vi "Function Generator Sweep.vi"(1 "Action":T3=enum."Identify", 2 "Parameters":variant) -> (6 "Output":variant, 7 "Stop":bool)   [LabVIEW 2020]
doc: "This VI reads a single reading from a Keithley 2001 multimeter. The stop boolean is always false. If no reading is obtained a single zero is returned.\nScott Hannahs, NHMFL-FSU, Nov 1993"
uses:
  Sub Controls/Instrument Actions.ctl
  Sub Controls/Instrument Match.ctl
  Sub Controls/Public.ctl
  Sub Controls/Scan Output.ctl
  Sub Controls/Instrument IDN.ctl
  Sub Controls/User Event Command.ctl
  <vilib>/Instr/_visa.llb/VISA GPIB Control REN Mode.ctl
panel:
  in  "Index":i32
  in  "Wait After Setting":dbl=5.0 format="%<%M:%S>t"
  in  "Mapping":bool
  in  "Time":dbl=1200.0 format="%<%H:%M:%S>t"
  in  "End Value":dbl=20.0
  in  "Start Value":dbl=1.0
  in  "Mode":bool
  out "Title":string
  in  "Public":T1
  in  "Address":u16(ring)
  out "Model":string
  in  "Instruments":T2[](array[typedef])=[{"Model"="DS360", "Manufacturer"="StanfordResearchSystems", "Term Character"="", "Wait Time (mS)"=0, "Wait for SRQ"=FALSE, "Type"="Func. Gen."}, {"Model"="SR830", "Manufacturer"="Stanford_Research_Systems", "Term Character"="", "Wait Time (mS)"=0, "Wait for SRQ"=FALSE, "Type"="Func. Gen."}, {"Model"="SR865A*", "Manufacturer"="Stanford_Research_Systems", "Term Character"="", "Wait Time (mS)"=0, "Wait for SRQ"=FALSE, "Type"="Func. Gen."}, {"Model"="SR860", "Manufacturer"="Stanford_Research_Systems", "Term Character"="", "Wait Time (mS)"=0, "Wait for SRQ"=FALSE, "Type"="Func. Gen."}]
  out "Measurement":dbl[](array[numeric]) format="%^_7e"
  in  "VISA resource name":refnum<visa-resource-name>
  # "Term Char"
  # "Wait Time (mS)"
  # "Wait for SRQ?"
  # "Type"
  # "Manufacturer"
  # "Model"
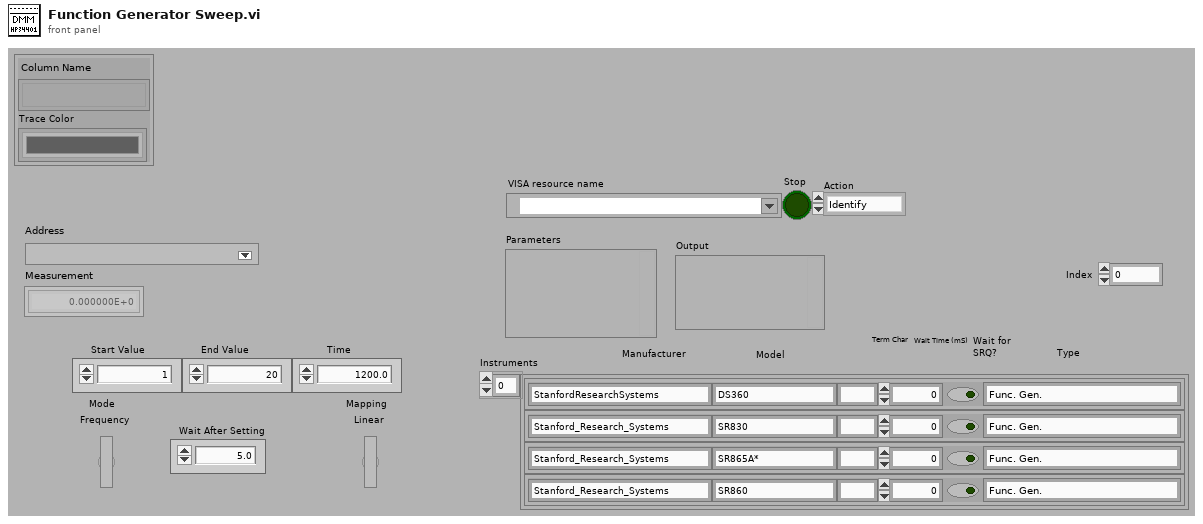
[diagram p1: front panel]
types:
  T1 = typedef "Public.ctl" = cluster{"Column Name":string[], "Trace Color":u32[]}
  T2 = typedef "Instrument Match.ctl" = cluster{"Model":string, "Manufacturer":string, "Term Character":string, "Wait Time (mS)":u32, "Wait for SRQ":bool, "Type":string}
  T3 = typedef "Instrument Actions.ctl" = enum16{"Scan", "Identify", "New", "Configure", "Initialize", "Test", "Read", "Close"}
  T4 = typedef "Scan Output.ctl" = cluster{"Manufacturer":string, "Model":string, "Info":string, "Revision":string, "error out":errorcluster}
  T5 = typedef "Instrument IDN.ctl" = cluster{"VISA Address":string, "Status":u16, "Manufacturer":string, "Model":string, "Info":string, "Info 2":string, "Misc Data":variant}
  T6 = typedef "User Event Command.ctl" = enum32{"Stop Config"}
  T7 = typedef "VISA GPIB Control REN Mode.ctl" = u16
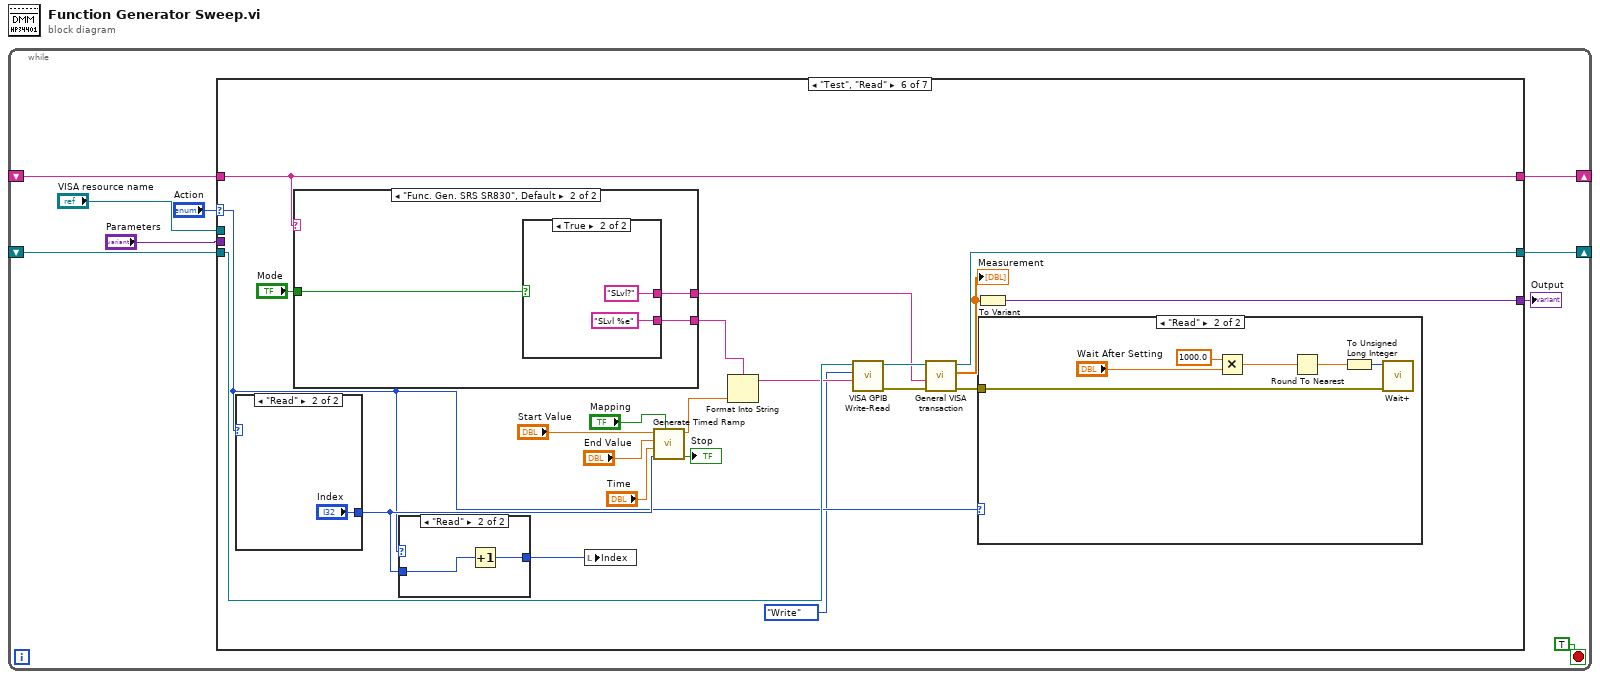
[diagram p0: block diagram]
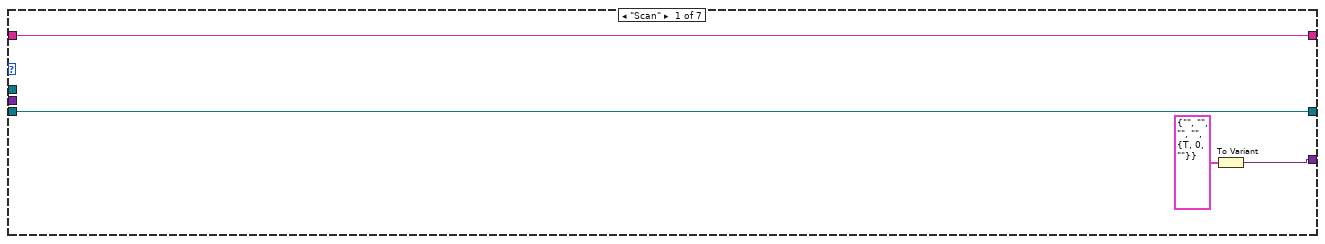
[diagram p2: hidden frame]
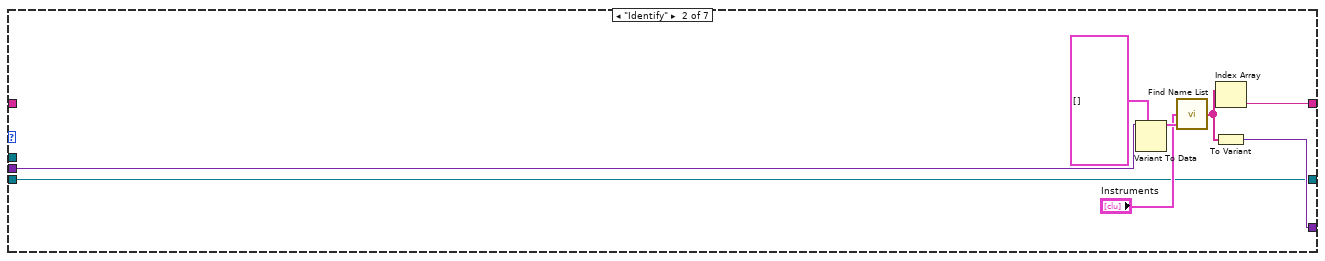
[diagram p3: hidden frame]
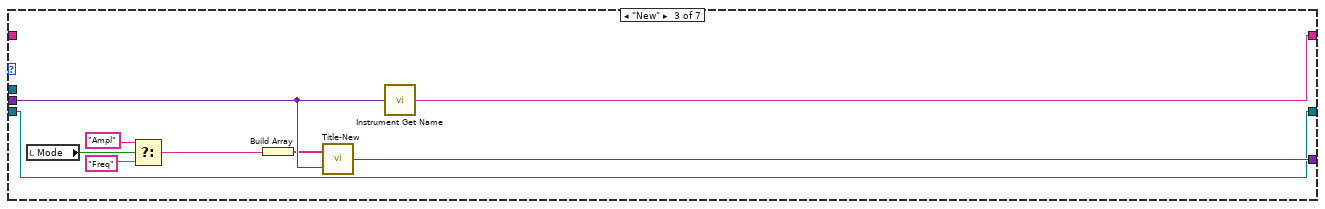
[diagram p4: hidden frame]
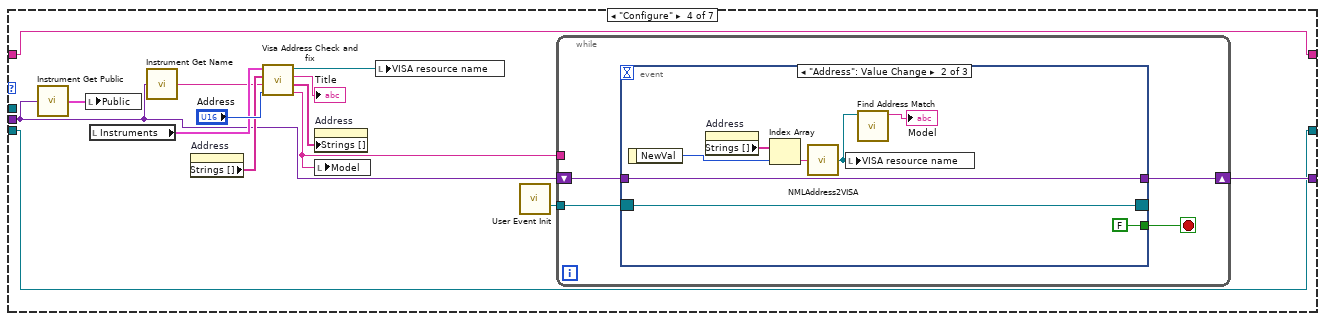
[diagram p5: hidden frame]
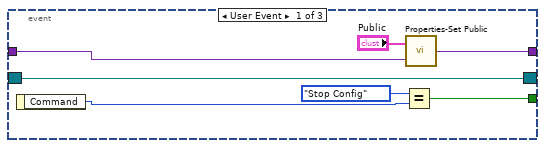
[diagram p6: hidden frame]
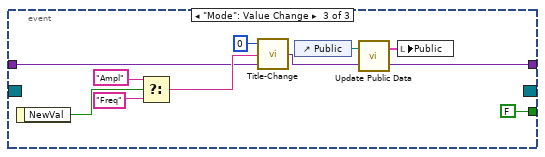
[diagram p7: hidden frame]
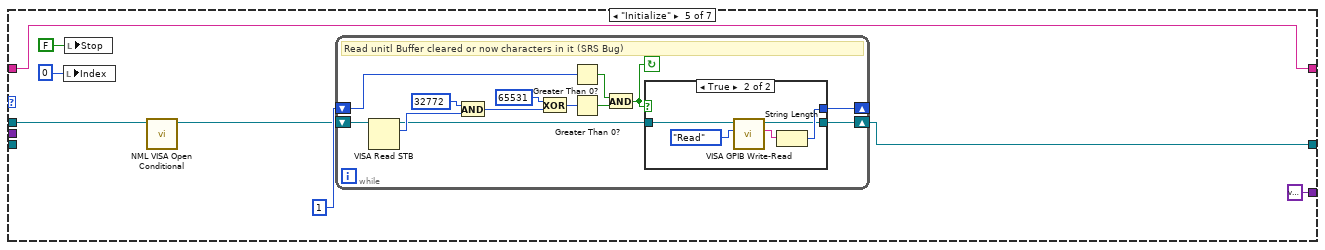
[diagram p8: hidden frame]
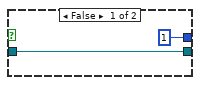
[diagram p9: hidden frame]
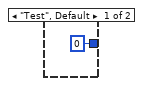
[diagram p12: hidden frame]
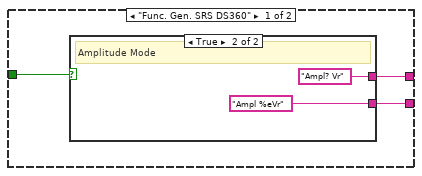
[diagram p13: hidden frame]
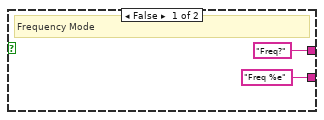
[diagram p14: hidden frame]
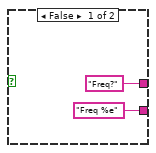
[diagram p15: hidden frame]
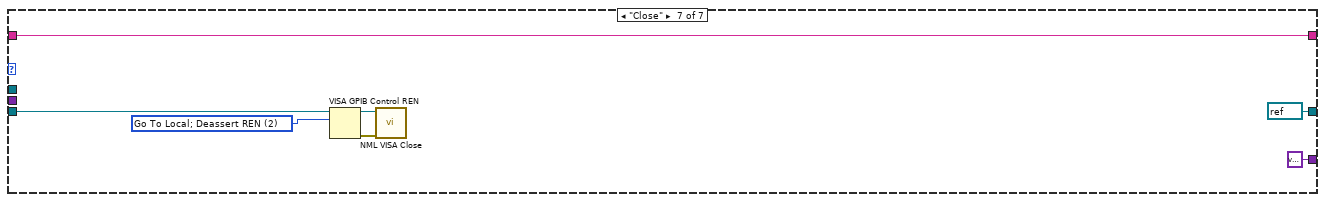
[diagram p16: hidden frame]
diagram:
  n1 = while {
    shift-right: [w5] -> _
    shift-left: _ -> [w4]
    shift-right: [w2] -> _
    shift-left: _ -> [w1]
    stop <- TRUE stop-if-true
    n2 = case shown="\"Test\", \"Read\"" "Action" {
      selector: "Action" -> [_ _ _ _ _ w109 _]
      tunnel: [w13 w21 w30 w38 variant ("Variant") w124 variant ("Variant")] -> w7
      tunnel: "VISA resource name" -> [_ _ _ _ w82 _ _]
      tunnel: [w12 w16 w26 w31 w80 w108 w153] -> w5
      tunnel: w4 -> [w12 _ _ w31 w80 w108 w153]
      tunnel: "Parameters" -> [_ w20 w28 w34 _ _ _]
      tunnel: [w11 w14 w29 w35 w75 w123 refnum<visa-resource-name> refnum ("Open VISA Resource name")] -> w2
      tunnel: w1 -> [w11 w14 w29 w35 _ w115 w150]
      frame "Scan" {
        n3 = To Variant(anything=T4 {"Manufacturer"="", "Model"="", "Info"="", "Revision"="", "error out"={"status"=TRUE, "code"=0, "source"=""}} ("Scan Output")) -> (Variant=w13:variant)
      }
      frame "Identify" {
        n4 = Variant To Data(type=T5[] [], Variant=w20) -> (data=w18:T5[])  [unwired: 1 in, 1 out]
        n5 = call "Find Name List.vi"("Bus Scan"=w18, "Instruments"="Instruments") -> ("Names"=w15:string[])  [unwired: 1 in]
        n6 = Index Array(array=w15) -> (element=w16:string)  [unwired: 1 in]
        n7 = To Variant(anything=w15) -> (Variant=w21:variant)
      }
      frame "New" {
        n8 = local read "Mode"() -> (w25:bool)
        n9 = Select(t="Ampl", s=w25, f="Freq") -> (s? t:f=w24:string)
        n10 = Build Array(w24) -> (w27:string[])
        n11 = call "Title-New.vi"("Parameters"=w28, "Array"=w27) -> ("Instrument Prop"=w30:variant)
        n12 = call "Instrument Get Name.vi"("Parameters"=w28) -> ("Type"=w26:string)
      }
      frame "Configure" {
        n13 = call "Instrument Get Public.vi"("Variant"=w34) -> ("Public"=w39:T1)
        n14 = local write "Public"(w39) -> ()
        n15 = local read "Instruments"() -> (w41:T2[])
        n16 = call "Instrument Get Name.vi"("Parameters"=w34) -> ("Type"=w33:string)
        n17 = property on="Address" class="Ring (strict)"() -> ("Strings []"=w42:string[])  [unwired: 2 in, 2 out]
        n18 = call "Visa Address Check and fix.vi"("Address"="Address", "Name"=w33, "NML Addresses"=w42, "Instruments"=w41) -> ("Model"=w40:string, "NML Addresses"=w44:string[], "Title"=→"Title":string, "VISA resource name"=w36:refnum<visa-resource-name>)  [unwired: 2 out]
        n19 = property on="Address" class="Ring (strict)"("Strings []"=w44) -> ()  [unwired: 2 in, 2 out]
        n20 = local write "Model"(w40) -> ()
        n21 = local write "VISA resource name"(w36) -> ()
        n22 = call "User Event Init.vi"() -> ("Event Registration Refnum"=w37:refnum<event-registration>)  [unwired: 14 in, 1 out]
        n23 = while {
          tunnel: w40 -> [_]
          tunnel: w37 -> [w45]
          shift-right: [w48] -> w38
          shift-left: w34 -> [w46]
          stop <- w47 stop-if-true
          n24 = event shown="[1] \"Address\": Value Change" {
            selector: w45 -> [w49 w57 _]
            dyn-events: [w49 w57 _] -> _
            timeout: _ -> [_ _ _]
            tunnel: [w53 w58 w66] -> w48
            tunnel: [w51 FALSE FALSE] -> w47
            tunnel: w46 -> [w54 w58 w69]
            event User Event {
              n25 = event-data() -> ("Command"=w55:T6)  [unwired: 1 in]
              n26 = Equal?(x=User_Event_Command."Stop Config", y=w55) -> (x = y?=w51:bool)
              n27 = call "Properties-Set Public.vi"("Variant"=w54, "New Public"="Public") -> ("Variant 2"=w53:variant)
            }
            event "Address": Value Change {
              n28 = event-data() -> ("NewVal"=w63:u16)  [unwired: 1 in]
              n29 = property on="Address" class="Ring (strict)"() -> ("Strings []"=w60:string[])  [unwired: 2 in, 2 out]
              n30 = Index Array(array=w60, index=w63) -> (element=w61:string)
              n31 = call "NMLAddress2VISA.vi"("NML Address"=w61) -> ("VISA resource name"=w56:refnum<visa-resource-name>)
              n32 = local write "VISA resource name"(w56) -> ()
              n33 = call "Find Address Match.vi"("VISA resource name"=w56) -> ("Model"=→"Model":string)  [unwired: 3 in, 3 out]
            }
            event "Mode": Value Change {
              n34 = event-data() -> ("NewVal"=w72:bool)  [unwired: 1 in]
              n35 = Select(t="Ampl", s=w72, f="Freq") -> (s? t:f=w71:string)
              n36 = call "Title-Change.vi"("Parameters"=w69, "New Title"=w71, "Index"=0) -> ("Variant"=w67:variant)
              n37 = control-ref of="Public"() -> (w64:refnum<vi>)
              n38 = call "Update Public Data.vi"("Variant In"=w67, "Public 2"=w64) -> ("Variant Out"=w66:variant, "Public"=w65:T1)
              n39 = local write "Public"(w65) -> ()
            }
          }
        }
      }
      frame "Initialize" {
        n40 = local write "Index"(0 ("Index")) -> ()
        n41 = local write "Stop"(FALSE ("Stop")) -> ()
        n42 = call "NML VISA Open Conditional.vi"("VISA resource name"=w82) -> ("dup VISA Session"=w76:refnum<visa-resource-name>)  [unwired: 8 in, 2 out]
        n43 = while {
          shift-right: [w87] -> w75
          shift-left: w76 -> [w86]
          shift-right: [w84] -> _
          shift-left: 1 -> [w85]
          stop <- w83 continue-if-true
          # "Read unitl Buffer cleared or now characters in it (SRS Bug)"
          n44 = VISA Read STB(11:w86) -> (2:w93:u16, 3:w92:refnum<visa-resource-name>)  [unwired: 1 in, 1 out]
          n45 = And(x=u16 32772, y=w93) -> (x .and. y?=w91:u16)
          n46 = Exclusive Or(1:w91, 2:u16 65531) -> (0:w95:u16)
          n47 = Greater Than 0?(x=w85) -> (x > 0?=w88:bool)
          n48 = Greater Than 0?(x=w95) -> (x > 0?=w94:bool)
          n49 = And(x=w88, y=w94) -> (x .and. y?=w83:bool)
          n50 = case shown="True" w83 {
            tunnel: w92 -> [w96 w99]
            tunnel: [1 w102] -> w84
            tunnel: [w96 w98] -> w87
            frame False {
            }
            frame True {
              n51 = call "VISA GPIB Write-Read.vi"("Action"=enum16{"Write", "Read", "Write & Read"}."Read", "VISA resource name"=w99) -> ("String Returned"=w101:string, "dup VISA Session"=w98:refnum<visa-resource-name>)  [unwired: 6 in, 2 out]
              n52 = String Length(string=w101) -> (length=w102:i32)
            }
          }
        }
      }
      frame "Test", "Read" {
        n53 = case shown="\"Read\"" w109 {
          tunnel: [0 ("Index") "Index"] -> w112
          frame "Test", Default {
          }
          frame "Read" {
          }
        }
        n54 = case shown="\"Func. Gen. SRS SR830\", Default" w108 {
          tunnel: [w137 w145] -> w105
          tunnel: "Mode" -> [w136 w144]
          tunnel: [w138 w143] -> w106
          frame "Func. Gen. SRS DS360" {
            n55 = case shown="True" w136 {
              tunnel: ["Freq %e" ("f") "Ampl %eVr"] -> w137
              tunnel: ["Freq?" ("f") "Ampl? Vr"] -> w138
              frame False {
                # "Frequency Mode"
              }
              frame True {
                # "Amplitude Mode"
              }
            }
          }
          frame "Func. Gen. SRS SR830", Default {
            n56 = case shown="True" w144 {
              tunnel: ["Freq %e" ("f") "SLvl %e"] -> w145
              tunnel: ["Freq?" ("f") "SLvl?"] -> w143
              frame False {
              }
              frame True {
              }
            }
          }
        }
        n57 = case shown="\"Read\"" w109 {
          tunnel: w112 -> [w131 w133]
          tunnel: [w131 w132] -> w111
          frame "Test", Default {
          }
          frame "Read" {
            n58 = Increment(x=w133) -> (x+1=w132:i32)
          }
        }
        n59 = local write "Index"(w111) -> ()
        n60 = call "Generate Timed Ramp.vi"("Log"="Mapping", "Point #"=w112, "Time (Hr:Min:Sec)"="Time", "Stop"="End Value", "Start"="Start Value") -> ("Stop"=→"Stop":bool, "Output"=w116:dbl)  [unwired: 2 out]
        n61 = Format Into String(format string=w105, w116) -> (resulting string=w104:string)  [unwired: 2 in, 1 out]
        n62 = call "VISA GPIB Write-Read.vi"("Command"=w104, "Action"=enum16{"Write", "Read", "Write & Read"}."Write", "VISA resource name"=w115) -> ("error out"=w113:errorcluster, "dup VISA Session"=w114:refnum<visa-resource-name>)  [unwired: 5 in, 2 out]
        n63 = call "General VISA transaction.vi"("error in (no error)"=w113, "Command String"=w106, "VISA Session"=w114) -> ("error out"=w110:errorcluster, "Measurement"=w122:dbl[], "dup VISA Session"=w123:refnum<visa-resource-name>)  [unwired: 3 in, 3 out]
        "Measurement" <- w122
        n64 = To Variant(anything=w122) -> (Variant=w124:variant)
        n65 = case shown="\"Read\"" w109 {
          tunnel: w110 -> [_ w130]
          frame "Test", Default {
          }
          frame "Read" {
            n66 = Multiply(x=1000.0, y="Wait After Setting") -> (x*y=w128:dbl)
            n67 = Round To Nearest(number=w128) -> (nearest integer value=w129:dbl)
            n68 = To Unsigned Long Integer(number=w129) -> (unsigned 32bit integer=w125:u32)
            n69 = call "Wait+.vi"("Error In"=w130, "milliseconds to wait"=w125) -> ()  [unwired: 4 in, 2 out]
          }
        }
      }
      frame "Close" {
        w152 = T7 2 items=["Deassert REN", "Assert REN", "Go To Local; Deassert REN ", "Assert REN; Address Device", "Local Lockout (Addressed Devices)", "Local Lockout (This Device)", "Go To Local"] ("Mode")
        n70 = VISA GPIB Control REN(10:w152, 11:w150) -> (0:w155:errorcluster, 3:w156:refnum<visa-resource-name>)  [unwired: 1 in]
        n71 = call "NML VISA Close.vi"("Error In"=w155, "VISA resource name"=w156) -> ()  [unwired: 9 in, 1 out]
      }
    }
    "Output" <- w7
  }
